vi "ChangeSampleRate.vi"(0 "object in":refnum<class "MTEC_Async.lvclass">, 2 "Sample Rate (Hz)":dbl format="%#_13g", 5 "error in (no error)":errorcluster) -> (14 "object out":refnum<class "MTEC_Async.lvclass">, 19 "error out":errorcluster)   [LabVIEW 2019, in "MTEC_Async.lvclass"]
uses:
  MTEC_Async.lvclass
  MTEC_Async.lvclass/MTEC_Async.ctl
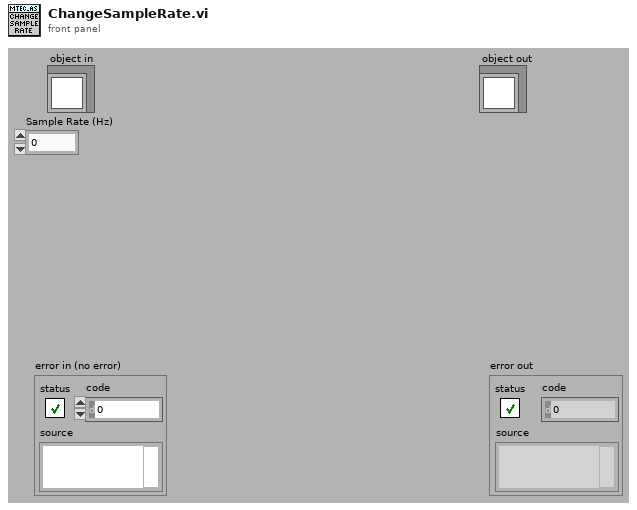
[diagram p1: front panel]
types:
  T1 = cluster{"Message":string, "Message Data":variant}
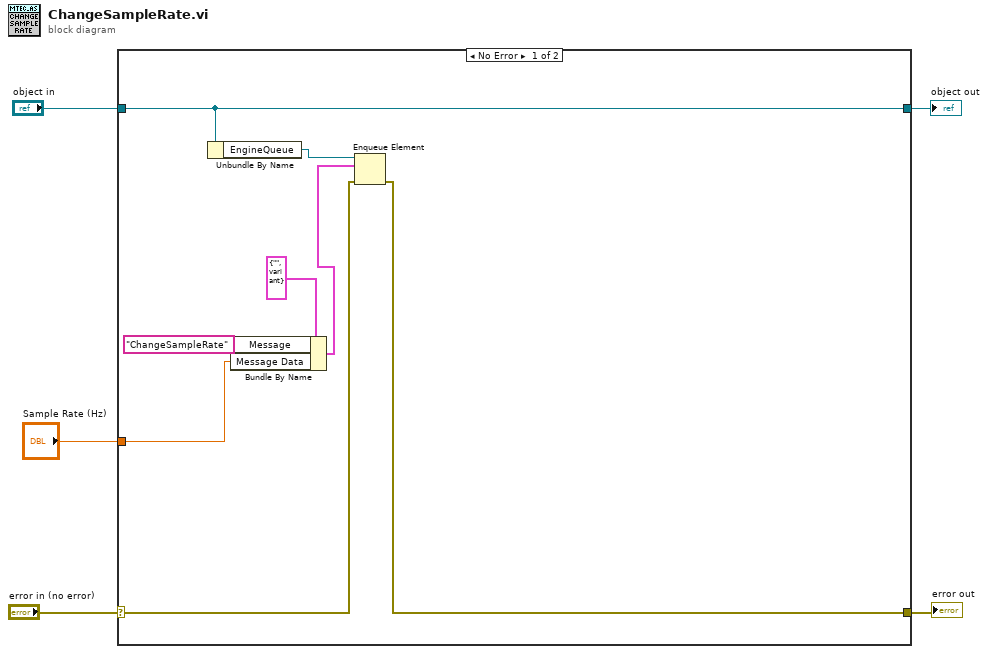
[diagram p0: block diagram]
diagram:
  n1 = case shown="No Error" "error in (no error)" {
    selector: "error in (no error)" -> [w7 w15]
    tunnel: [w6 w15] -> w4
    tunnel: [w13 w14] -> w2
    tunnel: "object in" -> [w13 w14]
    tunnel: "Sample Rate (Hz)" -> [w9 _]
    frame No Error {
      n2 = Unbundle By Name(w13) -> ("EngineQueue"=w12:refnum<queue>)
      n3 = Bundle By Name(cluster=T1 {"Message"="", "Message Data"=variant} ("element"), "Message"="ChangeSampleRate", "Message Data"=w9) -> (w8:T1)
      n4 = Enqueue Element(queue=w12, element=w8, error in (no error)=w7) -> (error out=w6:errorcluster)  [unwired: 1 in, 2 out]
    }
    frame Error {
    }
  }
  "error out" <- w4
  "object out" <- w2
